vi "Hardware List Updated.vi"(10 "error in (no error)":errorcluster, 11 "Hardware Update Data":T1) -> (2 "error out":errorcluster)   [LabVIEW 2020, in "RxnRover.lvlib"]
doc: "Fires the Update VI List Event with the provided Controller Array."
uses:
  RxnRover.lvlib
  Hardware Update Event Data.ctl
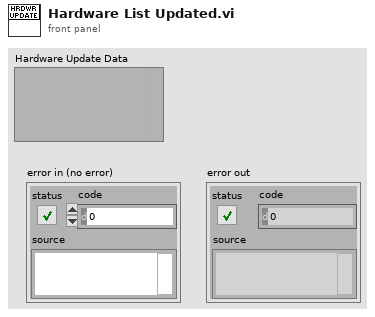
[diagram p1: front panel]
types:
  T1 = typedef "RxnRover.lvlib/Hardware Update Event Data.ctl" = variant
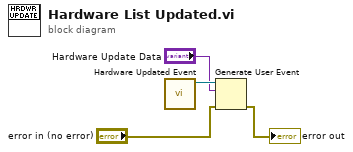
[diagram p0: block diagram]
diagram:
  n1 = call "Hardware Updated Event.vi"() -> ("Hardware Update Data"=w4:refnum<user-event>)  [unwired: 11 in]
  n2 = Generate User Event(user event=w4, event data cluster="Hardware Update Data", error in="error in (no error)") -> (error out=→"error out":errorcluster)  [unwired: 1 in, 1 out]
